vi "Blink_SDK_example.vi"() -> ()   [LabVIEW 2017]
uses:
  Blink_C_wrapper.dll
  ImageGen.dll
panel:
  out "ImgData 2":u8[](array[numeric])
  in  "Wait Timer":dbl=1000.0
  in  "Use External Triggers":bool
  out "BoardNum":i32
  out "ImgData":u8[](array[numeric])
  # "PCIe  LabVIEWSDK"
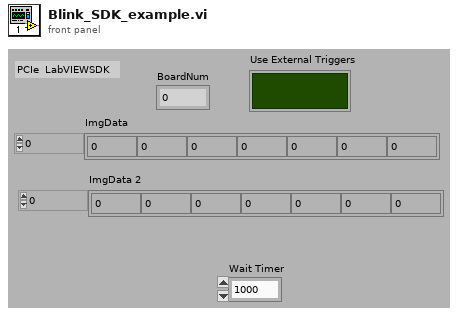
[diagram p1: front panel]
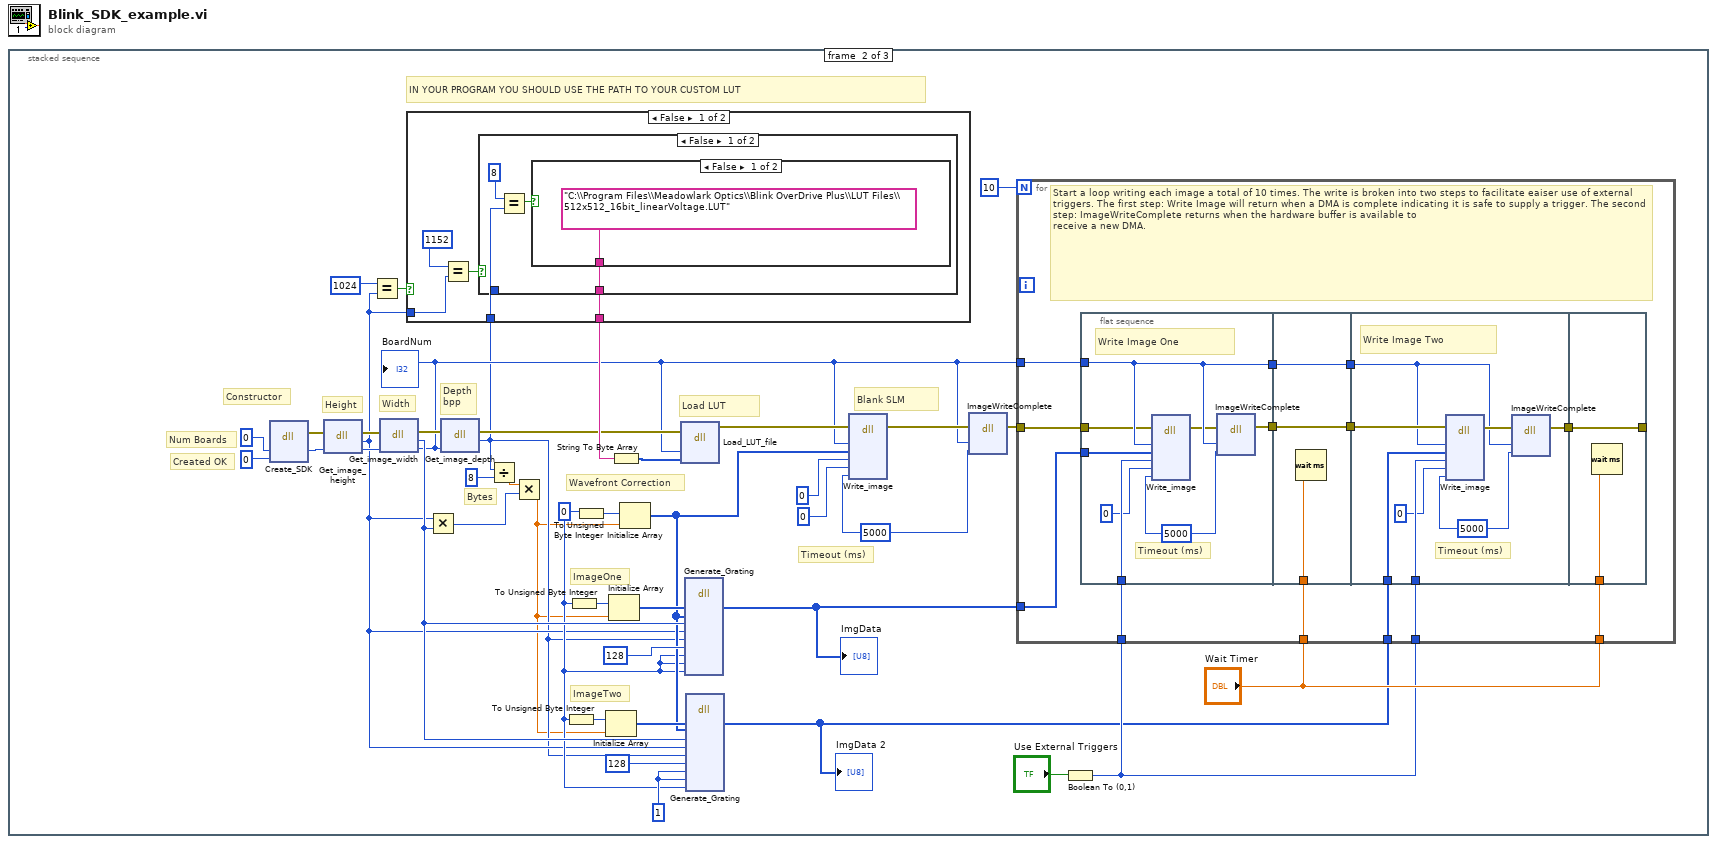
[diagram p0: block diagram]
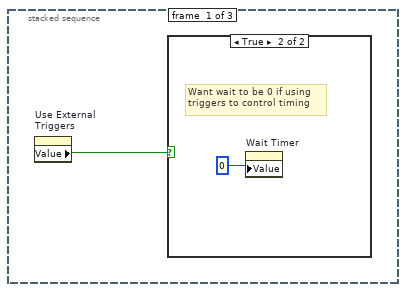
[diagram p2: hidden frame]
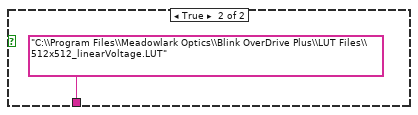
[diagram p4: hidden frame]
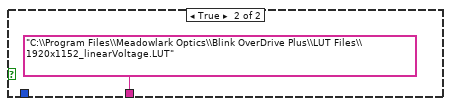
[diagram p5: hidden frame]
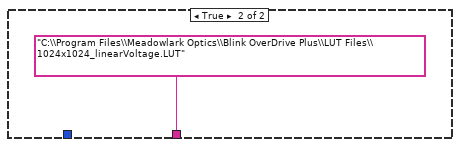
[diagram p6: hidden frame]
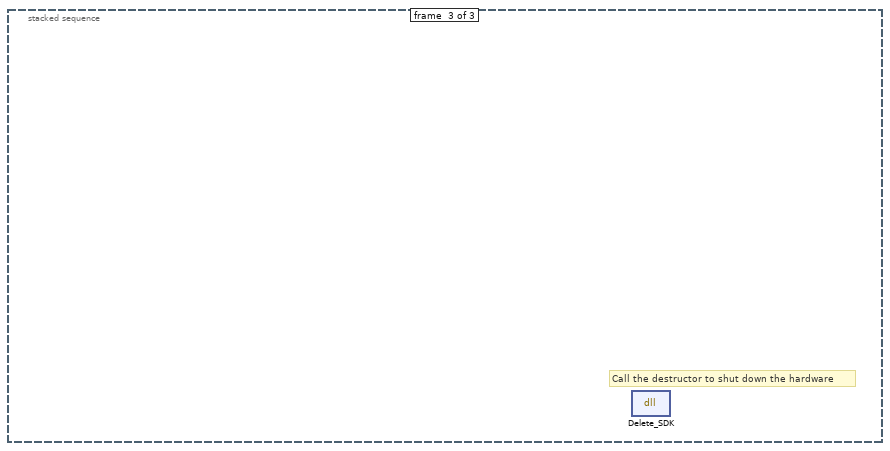
[diagram p7: hidden frame]
diagram:
  n1 = stacked-sequence {
    frame #0 {
      n2 = property on="Use External \nTriggers" class="Bool (strict)"() -> ("Value"=w1:bool)  [unwired: 2 in, 2 out]
      n3 = case shown="True" w1 {
        frame False {
        }
        frame True {
          # "Want wait to be 0 if using \ntriggers to control timing"
          n4 = property on="Wait Timer" class="DigNum (strict)"("Value"=0) -> ()  [unwired: 2 in, 2 out]
        }
      }
    }
    frame #1 {
      w23 = 5000
      w33 = 1
      w10 = 0
      # "Num Boards"
      # "Bytes"
      # "Depth\nbpp"
      # "Timeout (ms)"
      # "Blank SLM"
      # "IN YOUR PROGRAM YOU SHOULD USE THE PATH TO YOUR CUSTOM LUT"
      # "Load LUT"
      # "ImageTwo"
      # "ImageOne"
      # "Wavefront Correction"
      # "Width"
      # "Height"
      # "Created OK"
      # "Constructor"
      n5 = dll-call lib="C:/Meadowlark/Repos-git/MeadowlarkOverdrivePlus/src/Blink_SDK_example/Blink_C_wrapper.dll" fn="Create_SDK"("n_boards_found"=0, "constructed_ok"=0) -> (error out=w26:errorcluster, "n_boards_found"=w25:u64)  [unwired: 5 in, 1 out]
      n6 = dll-call lib="C:/Meadowlark/Repos-git/MeadowlarkOverdrivePlus/src/Blink_SDK_example/Blink_C_wrapper.dll" fn="Get_image_height"(error in=w26, "Board"=w25) -> (error out=w40:errorcluster, "return type"=w9:i32, "Board"=w41:u32)  [unwired: 2 in, 1 out]
      n7 = Equal?(x=1024, y=w9) -> (x = y?=w30:bool)
      n8 = dll-call lib="C:/Meadowlark/Repos-git/MeadowlarkOverdrivePlus/src/Blink_SDK_example/Blink_C_wrapper.dll" fn="Get_image_width"(error in=w40, "Board"=w41) -> (error out=w16:errorcluster, "return type"=w31:i32, "Board"=w14:u32)  [unwired: 2 in, 1 out]
      "BoardNum" <- w14
      n9 = Multiply(x=w9, y=w31) -> (x*y=w5:i32)
      n10 = dll-call lib="C:/Meadowlark/Repos-git/MeadowlarkOverdrivePlus/src/Blink_SDK_example/Blink_C_wrapper.dll" fn="Get_image_depth"(error in=w16, "Board"=w14) -> (error out=w15:errorcluster, "return type"=w7:i32)  [unwired: 3 in, 1 out]
      n11 = case shown="False" w30 {
        tunnel: [w45 "C:\\Program Files\\Meadowlark Optics\\Blink OverDrive Plus\\LUT Files\\1024x1024_linearVoltage.LUT"] -> w28
        tunnel: w9 -> [w48 _]
        tunnel: w7 -> [w46 _]
        frame False {
          n12 = Equal?(x=1152, y=w48) -> (x = y?=w47:bool)
          n13 = case shown="False" w47 {
            tunnel: [w50 "C:\\Program Files\\Meadowlark Optics\\Blink OverDrive Plus\\LUT Files\\1920x1152_linearVoltage.LUT"] -> w45
            tunnel: w46 -> [w52 _]
            frame False {
              n14 = Equal?(x=8, y=w52) -> (x = y?=w51:bool)
              n15 = case shown="False" w51 {
                tunnel: ["C:\\Program Files\\Meadowlark Optics\\Blink OverDrive Plus\\LUT Files\\512x512_16bit_linearVoltage.LUT" "C:\\Program Files\\Meadowlark Optics\\Blink OverDrive Plus\\LUT Files\\512x512_linearVoltage.LUT"] -> w50
                frame False {
                }
                frame True {
                }
              }
            }
            frame True {
            }
          }
        }
        frame True {
        }
      }
      n16 = Divide(x=w7, y=8) -> (x/y=w6:dbl)
      n17 = Multiply(x=w6, y=w5) -> (x*y=w4:dbl)
      n18 = To Unsigned Byte Integer(number=w10) -> (unsigned 8bit integer=w37:u8)
      n19 = To Unsigned Byte Integer(number=w10) -> (unsigned 8bit integer=w38:u8)
      n20 = To Unsigned Byte Integer(number=w10) -> (unsigned 8bit integer=w39:u8)
      n21 = Initialize Array(w37, w4) -> (w34:u8[])
      n22 = Initialize Array(w38, w4) -> (w36:u8[])
      n23 = String To Byte Array(string=w28) -> (unsigned byte array=w27:u8[])
      n24 = Initialize Array(w39, w4) -> (w13:u8[])
      n25 = dll-call lib="C:/Meadowlark/Repos-git/MeadowlarkOverdrivePlus/src/Blink_SDK_example/Blink_C_wrapper.dll" fn="Load_LUT_file"(error in=w15, "Board"=w14, "LUTPath"=w27) -> (error out=w21:errorcluster)  [unwired: 5 in, 1 out]
      n26 = dll-call lib="C:/Meadowlark/Repos-git/MeadowlarkOverdrivePlus/src/Blink_SDK_example/ImageGen.dll" fn="Generate_Grating"("Array"=w36, "WFC"=w13, "Width"=w31, "Height"=w9, "Depth"=w7, "Period"=128, "Increasing"=w10, "Horizontal"=w10, "RGB"=w10) -> ("Array"=w11:u8[])  [unwired: 12 in, 2 out]
      "ImgData" <- w11
      n27 = dll-call lib="C:/Meadowlark/Repos-git/MeadowlarkOverdrivePlus/src/Blink_SDK_example/ImageGen.dll" fn="Generate_Grating"("Array"=w34, "WFC"=w13, "Width"=w31, "Height"=w9, "Depth"=w7, "Period"=128, "Increasing"=w33, "Horizontal"=w33, "RGB"=w10) -> ("Array"=w12:u8[])  [unwired: 12 in, 2 out]
      "ImgData 2" <- w12
      n28 = dll-call lib="C:/Meadowlark/Repos-git/MeadowlarkOverdrivePlus/src/Blink_SDK_example/Blink_C_wrapper.dll" fn="Write_image"(error in=w21, "board"=w14, "Image"=w13, "WaitForTrigger"=0, "OutputPulseImageFlip"=0, "timeout"=w23) -> (error out=w22:errorcluster)  [unwired: 8 in, 1 out]
      n29 = dll-call lib="C:/Meadowlark/Repos-git/MeadowlarkOverdrivePlus/src/Blink_SDK_example/Blink_C_wrapper.dll" fn="ImageWriteComplete"(error in=w22, "board"=w14, "timeout"=w23) -> (error out=w20:errorcluster)  [unwired: 5 in, 1 out]
      n30 = Boolean To (0,1)(Boolean="Use External Triggers") -> (0, 1=w18:i16)
      n31 = for {
        N: 10 -> [_]
        tunnel: w14 -> [w70]
        tunnel: w12 -> [w69]
        tunnel: "Wait Timer" -> [w66]
        tunnel: "Wait Timer" -> [w65]
        tunnel: w20 -> [w61]
        tunnel: w11 -> [w60]
        tunnel: w18 -> [w59]
        tunnel: w18 -> [w58]
        # "Start a loop writing each image a total of 10 times. The write is broken into two steps to facilitate eaiser use of external triggers. The first step: Write Image will return when a DMA is complete indicating it is safe to supply a trigger. The second step: ImageWriteComplete returns when the hardware buffer is available to \nreceive a new DMA."
        n32 = flat-sequence {
          tunnel: w70 -> [w77]
          tunnel: w60 -> [w78]
          tunnel: [w77] -> w68
          tunnel: [w74] -> w63
          tunnel: w61 -> [w73]
          tunnel: w59 -> [w72]
          tunnel: w68 -> [w81]
          tunnel: [w81] -> w67
          tunnel: w66 -> [w80]
          tunnel: [w79] -> w64
          tunnel: w63 -> [w79]
          tunnel: w67 -> [w85]
          tunnel: w69 -> [w89]
          tunnel: w64 -> [w88]
          tunnel: [w86] -> w62
          tunnel: w58 -> [w83]
          tunnel: w65 -> [w91]
          tunnel: [w90] -> _
          tunnel: w62 -> [w90]
          frame #0 {
            w76 = 5000
            # "Timeout (ms)"
            # "Write Image One"
            n33 = dll-call lib="C:/Meadowlark/Repos-git/MeadowlarkOverdrivePlus/src/Blink_SDK_example/Blink_C_wrapper.dll" fn="Write_image"(error in=w73, "board"=w77, "Image"=w78, "WaitForTrigger"=w72, "OutputPulseImageFlip"=0, "timeout"=w76) -> (error out=w75:errorcluster)  [unwired: 8 in, 1 out]
            n34 = dll-call lib="C:/Meadowlark/Repos-git/MeadowlarkOverdrivePlus/src/Blink_SDK_example/Blink_C_wrapper.dll" fn="ImageWriteComplete"(error in=w75, "board"=w77, "timeout"=w76) -> (error out=w74:errorcluster)  [unwired: 5 in, 1 out]
          }
          frame #1 {
            n35 = Wait (ms)(milliseconds to wait=w80) -> ()  [unwired: 1 out]
          }
          frame #2 {
            w84 = 5000
            # "Timeout (ms)"
            # "Write Image Two"
            n36 = dll-call lib="C:/Meadowlark/Repos-git/MeadowlarkOverdrivePlus/src/Blink_SDK_example/Blink_C_wrapper.dll" fn="Write_image"(error in=w88, "board"=w85, "Image"=w89, "WaitForTrigger"=w83, "OutputPulseImageFlip"=0, "timeout"=w84) -> (error out=w87:errorcluster)  [unwired: 8 in, 1 out]
            n37 = dll-call lib="C:/Meadowlark/Repos-git/MeadowlarkOverdrivePlus/src/Blink_SDK_example/Blink_C_wrapper.dll" fn="ImageWriteComplete"(error in=w87, "board"=w85, "timeout"=w84) -> (error out=w86:errorcluster)  [unwired: 5 in, 1 out]
          }
          frame #3 {
            n38 = Wait (ms)(milliseconds to wait=w91) -> ()  [unwired: 1 out]
          }
        }
      }
    }
    frame #2 {
      # "Call the destructor to shut down the hardware"
      n39 = dll-call lib="C:/Meadowlark/Repos-git/MeadowlarkOverdrivePlus/src/Blink_SDK_example/Blink_C_wrapper.dll" fn="Delete_SDK"() -> ()  [unwired: 4 in, 2 out]
    }
  }
